vi "Template.Async.vi"(10 "Parameters":variant, 11 "Process":refnum<class "Process.lvclass">) -> ()   [LabVIEW 2026, in "Template.lvlib" / "Template.lvclass"]
uses:
  Template.lvclass
  <userlib>/NIVS Inline Async API (Express)/_VS Inline Async API (Express)/Process/Process.lvclass
  <userlib>/NIVS Inline Async API (Express)/_VS Inline Async API (Express)/Process/Process.lvclass/Process.ctl
  <userlib>/NIVS Inline Async API (Express)/_Data Access Engine (Express)/Access Type Classes/Read/Read.lvclass/Read.ctl
  <userlib>/NIVS Inline Async API (Express)/_Data Access Engine (Express)/Access Type Classes/Write/Write.lvclass/Write.ctl
  <userlib>/NIVS Inline Async API (Express)/_Data Access Engine (Express)/Data Access Engine (Express)/Methods/Read.Data.vi
  <userlib>/NIVS Inline Async API (Express)/_Data Access Engine (Express)/Data Access Engine (Express)/Methods/Write.Data.vi
  <userlib>/NIVS Inline Async API (Express)/_VS Inline Async API (Express)/Process/Data Member Access/Read Data Access.vi
  <userlib>/NIVS Inline Async API (Express)/_Data Access Engine (Express)/Access Type Classes/Read/Read.ProcessData.vi
  <userlib>/NIVS Inline Async API (Express)/_Data Access Engine (Express)/Access Type Classes/Write/Write.ProcessData.vi
  <userlib>/NIVS Inline Async API (Express)/_VS Inline Async API (Express)/Error Handling Process/SubVIs/Error.ConvertArray.vi
  <userlib>/NIVS Inline Async API (Express)/_Data Access Engine (Express)/Access Type Classes/Write/Write.Buffer.vi
  <userlib>/NIVS Inline Async API (Express)/_Data Access Engine (Express)/Access Type Classes/Write/Write.Commit.vi
  <userlib>/NIVS Inline Async API (Express)/_Data Access Engine (Express)/Data Access Engine (Express)/Methods/Write.Lookup.vi
  <userlib>/NIVS Inline Async API (Express)/_Data Access Engine (Express)/Data Access Engine (Express)/Methods/Read.Lookup.vi
  <userlib>/NIVS Inline Async API (Express)/_Data Access Engine (Express)/Data Access Engine (Express)/Data Access Engine (Express).lvclass
  Template.lvclass/Template.ctl
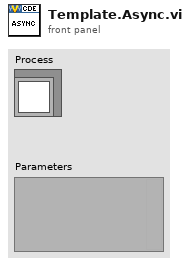
[diagram p1: front panel]
types:
  T1 = typedef "Data Access Engine (Express).lvlib/Data Access Engine (Express).lvclass/Write.DVR.ctl" = refnum<data-value>
  T2 = typedef "Data Access Engine (Express).lvlib/Data Access Engine (Express).lvclass/Read.DVR.ctl" = refnum<data-value>
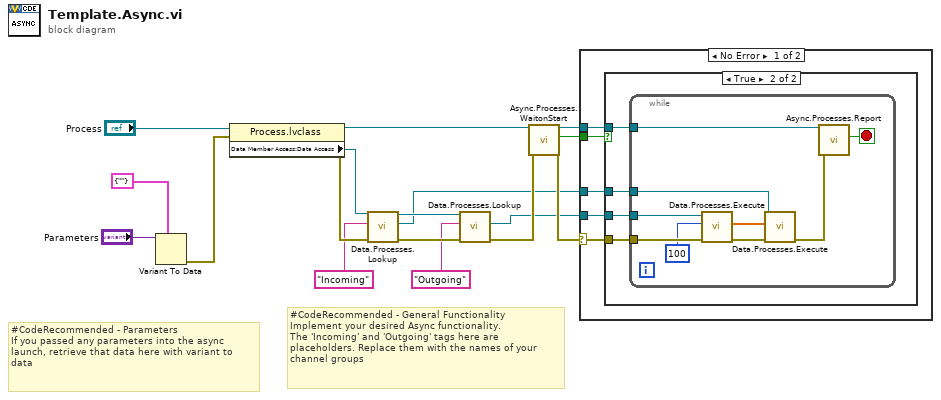
[diagram p0: block diagram]
diagram:
  # "#CodeRecommended - Parameters\nIf you passed any parameters into the async launch, retrieve that data here with variant to data"
  # "#CodeRecommended - General Functionality\nImplement your desired Async functionality.\nThe 'Incoming' and 'Outgoing' tags here are placeholders. Replace them with the names of your channel groups"
  n1 = Variant To Data(type=cluster{string} {""} ("TargetSettings"), Variant="Parameters") -> (error out=w3:errorcluster)  [unwired: 1 in, 1 out]
  n2 = property class="Process.lvclass"(reference="Process", error in=w3) -> (reference out=w10:refnum<class "Process.lvclass">, error out=w14:errorcluster, "Data Member Access:Data Access"=w12:refnum<class "Data Access Engine (Express).lvclass">)
  n3 = call-poly <userlib>:"Data.Processes.Lookup.vi"("error in"=w14, "Name"="Incoming", "Data Access API in"=w12) -> ("error out"=w15:errorcluster, "Ref"=w7:T1, "Data Access API out"=w11:refnum<class "Data Access Engine (Express).lvclass">)  [unwired: 5 in, 1 out]
  n4 = call-poly <userlib>:"Data.Processes.Lookup.vi"("error in"=w15, "Name"="Outgoing", "Data Access API in"=w11) -> ("error out"=w17:errorcluster, "Ref"=w8:T2)  [unwired: 5 in, 2 out]
  n5 = call <userlib>:"Async.Processes.WaitonStart.vi"("error in"=w17, "Process in"=w10) -> ("error out"=w16:errorcluster, "Execute"=w9:bool, "Process out"=w6:refnum<class "Process.lvclass">)  [unwired: 7 in]
  n6 = case shown="No Error" w16 {
    selector: w16 -> [w22 _]
    tunnel: w9 -> [w21 _]
    tunnel: w8 -> [w20 _]
    tunnel: w7 -> [w19 _]
    tunnel: w6 -> [w18 _]
    frame No Error {
      n7 = case shown="True" w21 {
        tunnel: w22 -> [_ w26]
        tunnel: w20 -> [_ w25]
        tunnel: w19 -> [_ w24]
        tunnel: w18 -> [_ w23]
        frame False {
        }
        frame True {
          n8 = while {
            tunnel: w26 -> [w35]
            tunnel: w25 -> [w32]
            tunnel: w24 -> [w30]
            tunnel: w23 -> [w28]
            stop <- w27 stop-if-true
            n9 = call-poly <userlib>:"Data.Processes.Execute.vi"("error in"=w35, "timeout ms"=100, "Ref"=w32) -> ("error out"=w34:errorcluster, "Values"=w29:dbl[])  [unwired: 6 in, 1 out]
            n10 = call-poly <userlib>:"Data.Processes.Execute.vi"("error in"=w34, "Values"=w29, "Ref"=w30) -> ("error out"=w33:errorcluster)  [unwired: 8 in]
            n11 = call <userlib>:"Async.Processes.Report.vi"("error in"=w33, "Process in"=w28) -> ("Stop"=w27:bool)  [unwired: 8 in, 1 out]
          }
        }
      }
    }
    frame Error {
    }
  }
